vi "IIR Filter.vi"(10 "Filter Power":dbl, 11 "Value":dbl) -> (3 "Filtered Value":dbl)   [LabVIEW 2015]
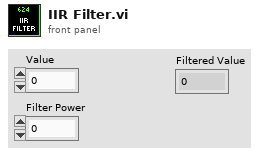
[diagram p1: front panel]
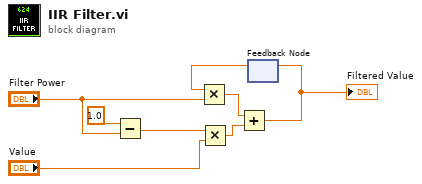
[diagram p0: block diagram]
diagram:
  n1 = Subtract(x=1.0, y="Filter Power") -> (x-y=w3:dbl)
  n2 = Multiply(x=w3, y="Value") -> (x*y=w2:dbl)
  n3 = feedback #1() -> (w6:dbl)  [unwired: 1 in]
  n4 = Multiply(x=w6, y="Filter Power") -> (x*y=w5:dbl)
  n5 = Add(x=w5, y=w2) -> (x+y=w4:dbl)
  "Filtered Value" <- w4
  n6 = feedback-in #1(w4) -> ()
